vi "Digital Write 1 Channel.vi"(7 "DAQ Module":i32, 8 "error constant":errorcluster, 9 "Value":bool=TRUE, 10 "Channel":i32, 11 "I-O.lvclass":refnum<class "I-O.lvclass">) -> (0 "error IO":errorcluster, 3 "I-O.lvclass 2":refnum<class "I-O.lvclass">)   [LabVIEW 2016, in "I-O.lvclass"]
uses:
  I-O.lvclass
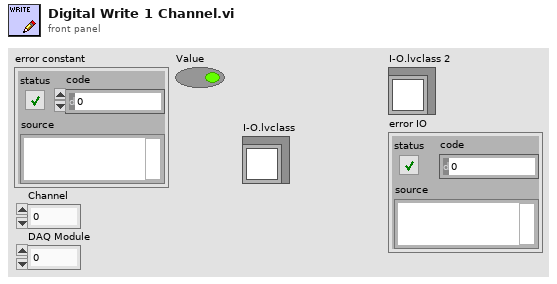
[diagram p1: front panel]
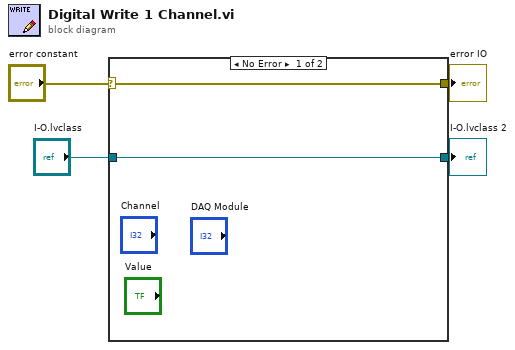
[diagram p0: block diagram]
diagram:
  n1 = case shown="No Error" "error constant" {
    selector: "error constant" -> [w6 w8]
    tunnel: [w6 w8] -> w3
    tunnel: [w5 w7] -> w2
    tunnel: "I-O.lvclass" -> [w5 w7]
    frame No Error {
    }
    frame Error {
    }
  }
  "I-O.lvclass 2" <- w2
  "error IO" <- w3
